vi "SCCSup Is File in LLB.vi"(11 "Path":path) -> (1 "is in LLB?":bool, 3 "converted path":path)   [LabVIEW 2017]
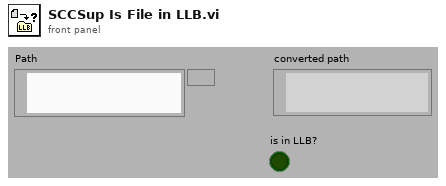
[diagram p1: front panel]
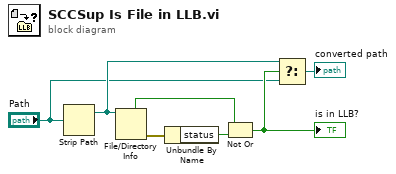
[diagram p0: block diagram]
diagram:
  n1 = Strip Path(path="Path") -> (stripped path=w3:path)  [unwired: 1 out]
  n2 = File/Directory Info(path=w3) -> (directory=w5:bool, error out=w7:errorcluster)  [unwired: 1 in, 5 out]
  n3 = Unbundle By Name(w7) -> ("status"=w6:bool)
  n4 = Not Or(1:w6, 2:w5) -> (0:w4:bool)
  "is in LLB?" <- w4
  n5 = Select(t=w3, s=w4, f="Path") -> (s? t:f=→"converted path":path)
